vi "PID Intake.vi"(8 "Cluster 3":T2={"Left Encoder"="Talon1", "Right Encoder"="Talon4", "Gyro Refnum"="Gyro", "Device Number"=enum."Dev0", "Right Refnum"="Talon5", "Left Refnum"="Talon2", "Right Intake"="Talon9", "Left Intake"="Talon7"}, 9 "Timeout":i16, 10 "Target Distance":dbl format="%#_13g", 11 "Target Angle":dbl) -> (0 "Cluster 2":T2={"Left Encoder"="Talon1", "Right Encoder"="Talon4", "Gyro Refnum"="Gyro", "Device Number"=enum."Dev0", "Right Refnum"="Talon5", "Left Refnum"="Talon2", "Right Intake"="Talon9", "Left Intake"="Talon7"})   [LabVIEW 2017]
uses:
  <vilib>/Rock Robotics/WPI/ThirdParty/Sensors/navX/_TypeDefs/FRIC_navX_DeviceNumbersTypeDef.ctl
  Public/Documents/Cross The Road Electronics/Phoenix-LabVIEW/Motor Controller/Controls/CTRE_Phoenix_MotorControl_ControlMode.ctl
  <vilib>/Rock Robotics/WPI/ThirdParty/Phoenix-LabVIEW/Motor Controller/Get/CTRE_Phoenix_MotorController_GetQuadratureData.vi
  <vilib>/addons/control/pid/pid.llb/PID (DBL).vi
  <vilib>/addons/control/pid/NI_PID_pid.lvlib
panel:
  out "In Range":dbl
  out "A-Setpoint":dbl
  in  "D - Lower Limit":dbl=-0.7 format="%#_13g"
  in  "D - Upper Limit":dbl=0.7 format="%#_13g"
  in  "A - Lower Limit":dbl=-1.0 format="%#_13g"
  in  "A - Upper Limit":dbl=1.0 format="%#_13g"
  out "D - Low Threshold":dbl
  out "D - High Threshold":dbl
  out "Cluster":cluster{dbl, dbl}
  out "Angle Modifier":dbl format="%.2f"
  out "Distance Modifier":dbl format="%.2f"
  out "Quadrature Position 4":i32
  out "Quadrature Position 1":i32
  out "Elapsed Time":u32
  out "Distance":i32
  out "Angle":dbl
  in  "A-D":dbl=0.001 format="%#_13g"
  in  "A-I":dbl format="%#_13g"
  in  "A-P":dbl=0.075 format="%#_13g"
  out "Right":dbl
  out "Left":dbl
  in  "D-P":dbl=5e-05 format="%#_13g"
  in  "D-I":dbl format="%#_13g"
  in  "D-D":dbl=1e-07 format="%#_13g"
  out "error out":errorcluster
  in  "error in":errorcluster
  # "pos 1-pos8=distance"
  # "Miami Valley\nDistance\n3E-5\n0\n.001\n.7\n-.7\n\nAngle\n.075\n0\n0\n.5\n-.5\n\n25k=20\" 20.25\"\n50k=39.75\"\n100k=78.5\"\n150k=116.5"
  # ".0002"
  # "4"
  # "2.5E-5"
  # "ALPHA encoders\nTalon1\nTalon4\n\nALPHA drive\nTalon2\nTalon5"
  # ".00001"
  # ".0005"
  # "8e-5/0/1e-7"
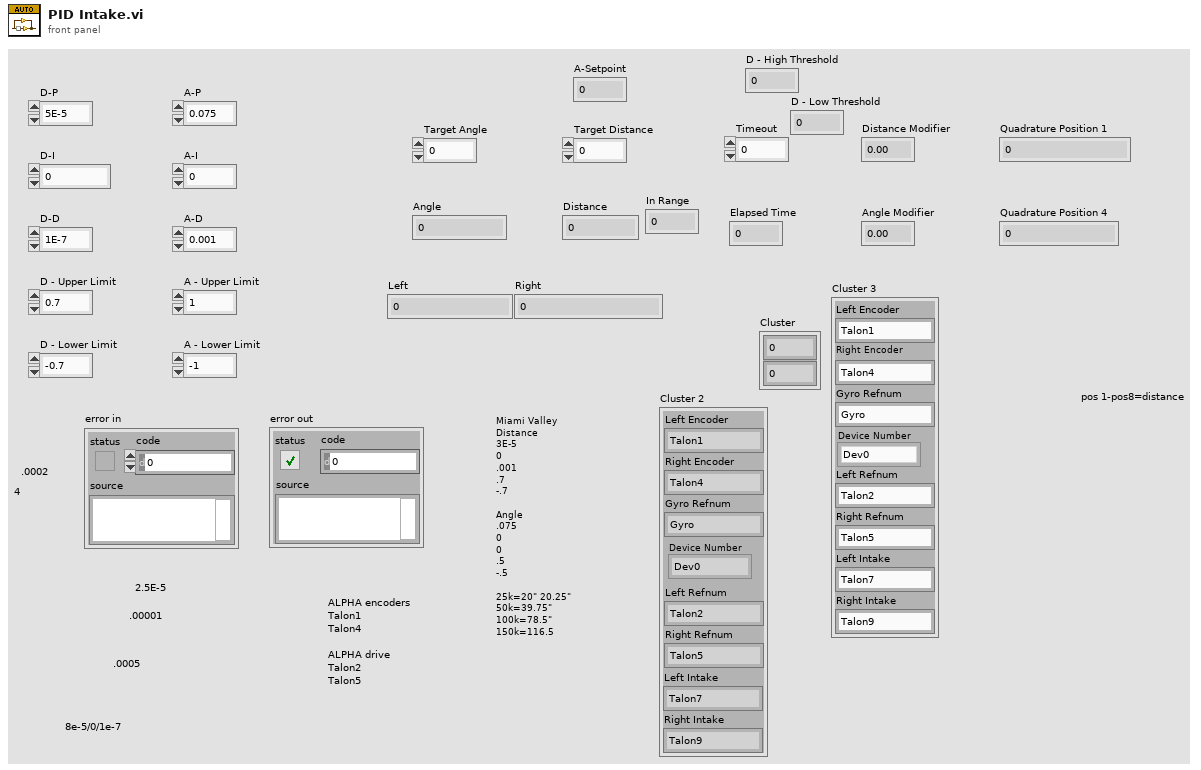
[diagram p1: front panel]
types:
  T1 = typedef "FRIC_navX_DeviceNumbersTypeDef.ctl" = enum16{"Dev0", "Dev1", "Dev2", "Dev3"}
  T2 = cluster{"Left Encoder":string, "Right Encoder":string, "Gyro Refnum":string, "Device Number":T1, "Right Refnum":string, "Left Refnum":string, "Right Intake":string, "Left Intake":string}
  T3 = typedef "CTRE_Phoenix_MotorControl_ControlMode.ctl" = u16
  T4 = typedef "WPI_GyroDevRef.ctl" = cluster{"DevStatus":errorcluster, "Analog Channel":T5, "Gain (VoltsPerDegree/Second)":dbl, "Gyro Type":enum16{"Analog", "XRS450"}, "Handle":i32, "SPI Bus":T6, "Device Found":bool, "Sample Rate":dbl, "Calibrate On Open":bool, "Offset":dbl}
  T5 = typedef "FPGA_AIChannel.ctl" = enum8{"AI 0", "AI 1", "AI 2", "AI 3", "AI MXP 0", "AI MXP 1", "AI MXP 2", "AI MXP 3", "Invalid"}
  T6 = typedef "spi_bus.ctl" = enum16{"SPI On-Board, CS0", "SPI On-Board, CS1", "SPI On-Board, CS2", "SPI On-Board, CS3", "SPI MXP", "Invalid"}
  T7 = typedef "WPI_MotorControlDeviceRef.ctl" = cluster{"DeviceStatus":errorcluster, "Type":T8, "PWM":cluster{"PWM Channel":T9, "DeadBand":T10}, "CAN":cluster{"Device Number":u8, "SetOutput VI Ref":variant, "GetOutput VI Ref":variant, "Enable VI Ref":variant, "Disable VI Ref":variant, "Data":variant}, "Invert":bool, "DIO PWM":cluster{"PWM \"Enable\" Channel":T9, "DIOChannel":T11, "PWM Rate":dbl}}
  T8 = typedef "WPI_MotorControlType.ctl" = enum16{"PWM", "CAN", "DIO PWM"}
  T9 = typedef "FPGA_DIOPWMChannel.ctl" = enum8{"PWM 0", "PWM 1", "PWM 2", "PWM 3", "PWM 4", "PWM 5", "PWM 6", "PWM 7", "PWM 8", "PWM 9", "PWM MXP 0", "PWM MXP 1", "PWM MXP 2", "PWM MXP 3", "PWM MXP 4", "PWM MXP 5", "PWM MXP 6", "PWM MXP 7", "PWM MXP 8", "PWM MXP 9", "Invalid"}
  T10 = typedef "WPI_PWMDeadband.ctl" = cluster{"Name":string, "maxPositivePwm":i32, "minPositivePwm":i32, "centerPwm":i32, "maxNegativePwm":i32, "minNegativePwm":i32, "angularRange":u16}
  T11 = typedef "FPGA_DIOChannel.ctl" = enum8{"DIO 0", "DIO 1", "DIO 2", "DIO 3", "DIO 4", "DIO 5", "DIO 6", "DIO 7", "DIO 8", "DIO 9", "DIO MXP 0", "DIO MXP 1", "DIO MXP 2", "DIO MXP 3", "DIO MXP 4", "DIO MXP 5", "DIO MXP 6", "DIO MXP 7", "DIO MXP 8", "DIO MXP 9", "DIO MXP 10", "DIO MXP 11", "DIO MXP 12", "DIO MXP 13", "DIO MXP 14", "DIO MXP 15", "SPI Port CS1", "SPI Port CS2", "SPI Port CS3", "SPI Port MISO", "SPI Port MOSI", "Invalid"}
  T12 = cluster{"D - Upper Limit":dbl, "D - Lower Limit":dbl}
  T13 = cluster{"A - Upper Limit":dbl, "A - Lower Limit":dbl}
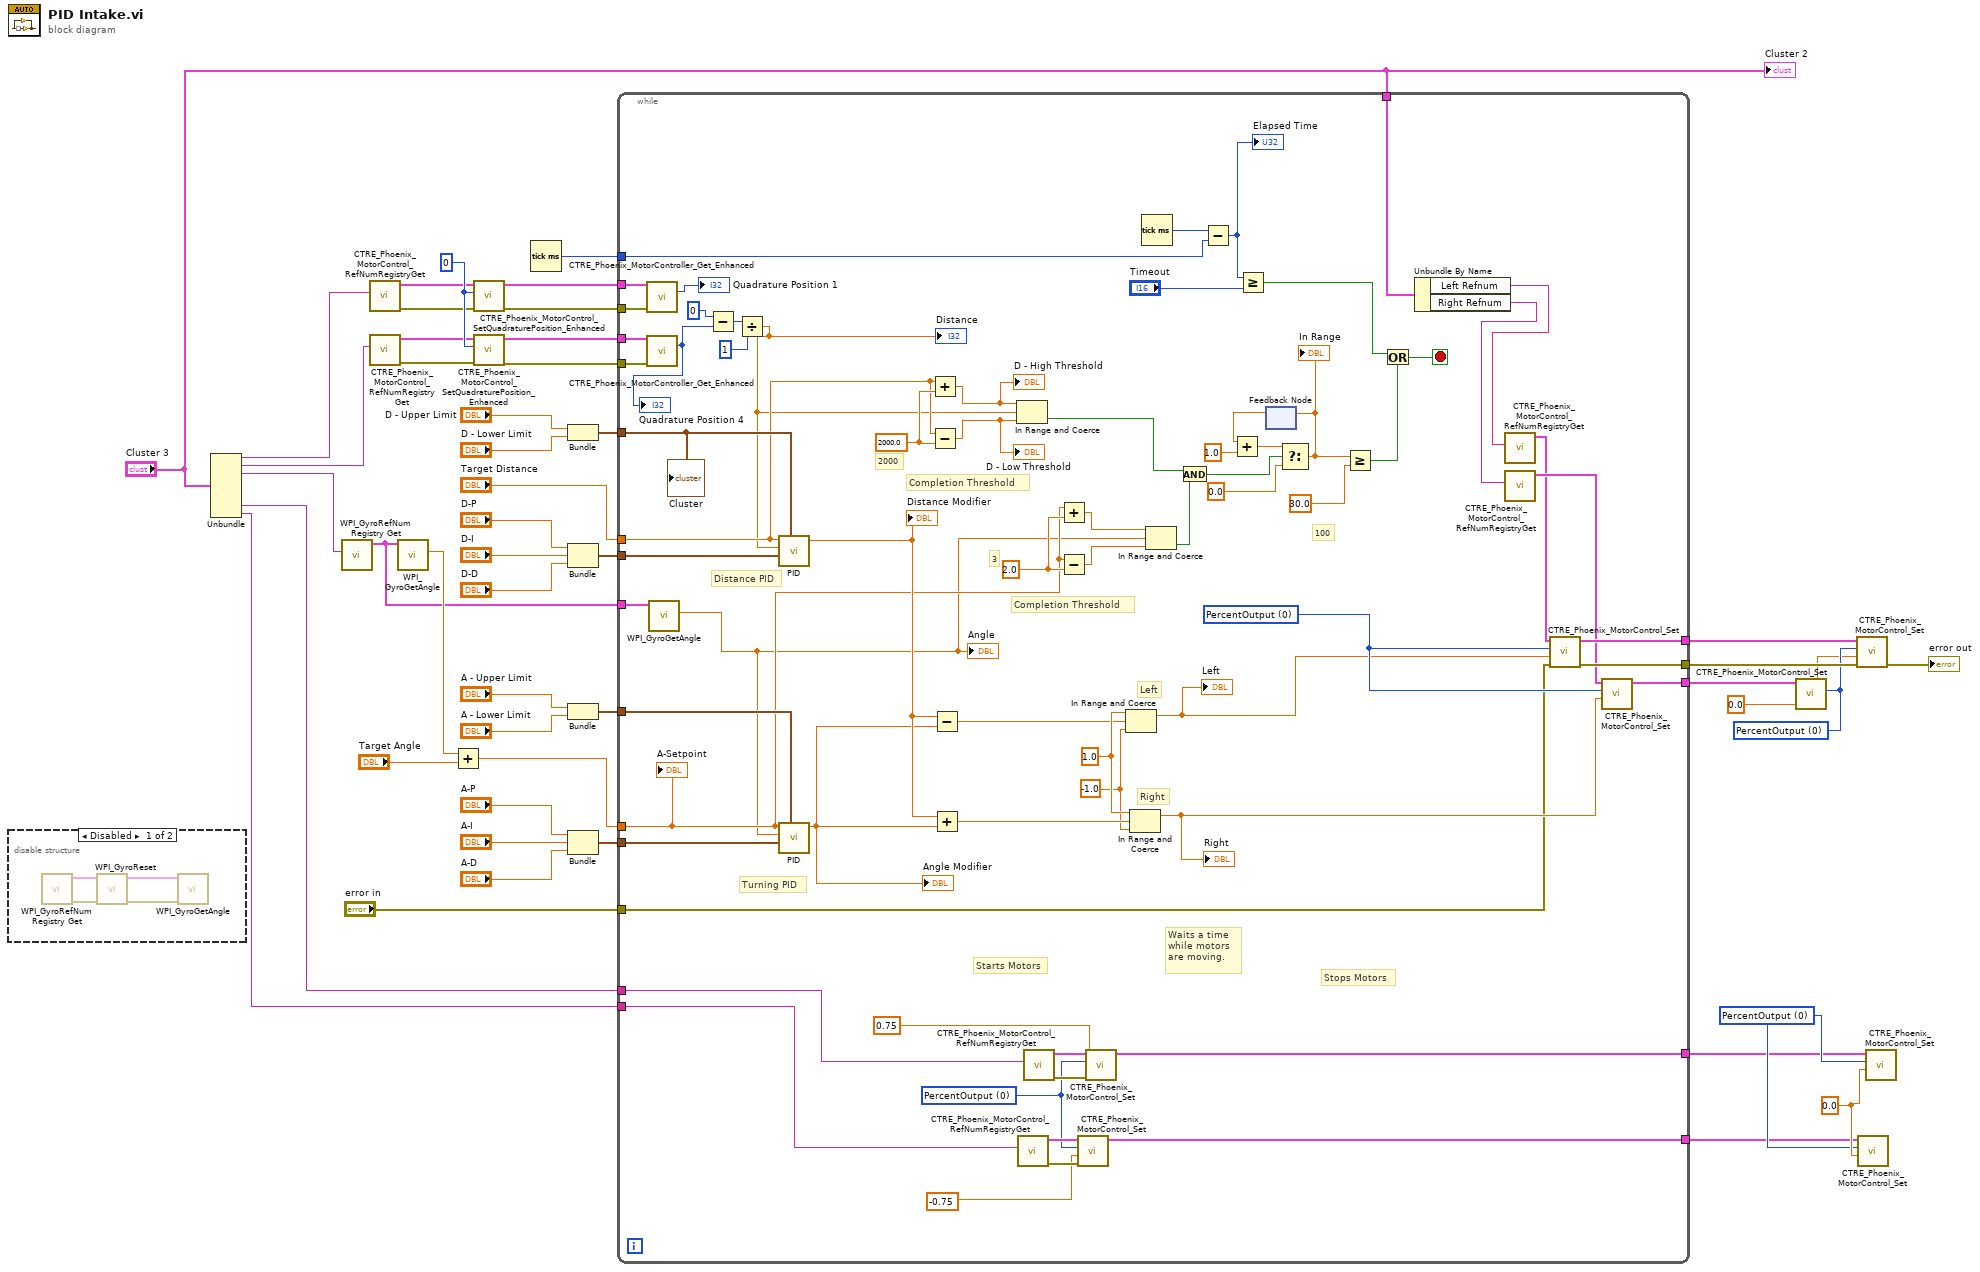
[diagram p0: block diagram]
diagram:
  w4 = 0.0 ("Output")
  w3 = T3 0 items=["PercentOutput"=0, "Position"=1, "Velocity"=2, "Current"=3, "Follower"=5, "MotionProfile"=6, "MotionMagic"=7, "MotionMagicArc"=8, "MotionProfileArc"=10, "Disabled"=15] ("Control Mode")
  w9 = 0.0 ("Output")
  w10 = T3 0 items=["PercentOutput"=0, "Position"=1, "Velocity"=2, "Current"=3, "Follower"=5, "MotionProfile"=6, "MotionMagic"=7, "MotionMagicArc"=8, "MotionProfileArc"=10, "Disabled"=15] ("Control Mode")
  w29 = 0 ("New Position")
  n1 = disable-structure shown="Disabled" {
    frame Disabled {
      n2 = call <vilib>:"WPI_GyroRefNum Registry Get.vi"() -> ("error out"=w49:errorcluster, "GyroDevRef"=w50:T4)  [unwired: 10 in]
      n3 = call <vilib>:"WPI_GyroReset.vi"("error in"=w49, "GyroDevRef"=w50) -> ("error out"=w47:errorcluster, "GyroDevRef"=w48:T4)  [unwired: 8 in]
      n4 = call <vilib>:"WPI_GyroGetAngle.vi"("error in"=w47, "GyroDevRef"=w48) -> ()  [unwired: 5 in, 5 out]
    }
    frame Enabled {
    }
  }
  n5 = Unbundle("Cluster 3") -> ("Left Encoder"=w23:string, "Right Encoder"=w22:string, "Gyro Refnum"=w19:string, "Right Intake"=w6:string, "Left Intake"=w5:string)  [unwired: 3 out]
  n6 = call <vilib>:"WPI_GyroRefNum Registry Get.vi"("refnum name"=w19) -> ("GyroDevRef"=w17:T4)  [unwired: 9 in, 1 out]
  n7 = call "CTRE_Phoenix_MotorControl_RefNumRegistryGet.vi"("refnum name"=w23) -> ("error out"=w25:errorcluster, "PhoenixMotorControlDevRef"=w16:T7)  [unwired: 9 in]
  n8 = call "CTRE_Phoenix_MotorControl_RefNumRegistryGet.vi"("refnum name"=w22) -> ("error out"=w27:errorcluster, "PhoenixMotorControlDevRef"=w15:T7)  [unwired: 9 in]
  n9 = call <vilib>:"WPI_GyroGetAngle.vi"("GyroDevRef"=w17) -> ("Angle"=w18:dbl)  [unwired: 6 in, 4 out]
  n10 = Add(x=w18, y="Target Angle") -> (x+y=w20:dbl)
  n11 = call "CTRE_Phoenix_MotorControl_SetQuadraturePosition_Enhanced.vi"("error in (no error)"=w25, "New Position"=w29, "PhoenixMotorControlDevRef"=w16) -> ("error out"=w26:errorcluster, "PhoenixMotorControlDevRef"=w31:T7)  [unwired: 7 in]
  n12 = call "CTRE_Phoenix_MotorControl_SetQuadraturePosition_Enhanced.vi"("error in (no error)"=w27, "New Position"=w29, "PhoenixMotorControlDevRef"=w15) -> ("error out"=w28:errorcluster, "PhoenixMotorControlDevRef"=w30:T7)  [unwired: 7 in]
  n13 = Tick Count (ms)() -> (millisecond timer value=w24:u32)
  n14 = Bundle("D - Upper Limit"="D - Upper Limit", "D - Lower Limit"="D - Lower Limit") -> (w44:T12)  [unwired: 1 in]
  n15 = Bundle("D-P"="D-P", "D-I"="D-I", "D-D"="D-D") -> (w33:cluster{"D-P":dbl, "D-I":dbl, "D-D":dbl})  [unwired: 1 in]
  n16 = Bundle("A - Upper Limit"="A - Upper Limit", "A - Lower Limit"="A - Lower Limit") -> (w41:T13)  [unwired: 1 in]
  n17 = Bundle("A-P"="A-P", "A-I"="A-I", "A-D"="A-D") -> (w37:cluster{"A-P":dbl, "A-I":dbl, "A-D":dbl})  [unwired: 1 in]
  n18 = while {
    tunnel: w44 -> [w119]
    tunnel: w41 -> [w117]
    tunnel: w37 -> [w113]
    tunnel: w33 -> [w112]
    tunnel: "Target Distance" -> [w100]
    tunnel: w20 -> [w93]
    tunnel: w30 -> [w110]
    tunnel: w31 -> [w109]
    tunnel: w28 -> [w108]
    tunnel: w26 -> [w107]
    tunnel: w24 -> [w104]
    tunnel: w17 -> [w83]
    tunnel: [w78] -> w14
    tunnel: [w77] -> w12
    tunnel: [w76] -> w11
    tunnel: "Cluster 3" -> [w75]
    tunnel: "error in" -> [w66]
    tunnel: w6 -> [w56]
    tunnel: w5 -> [w55]
    tunnel: [w52] -> w2
    tunnel: [w51] -> w1
    stop <- w88 stop-if-true
    w57 = T3 0 items=["PercentOutput"=0, "Position"=1, "Velocity"=2, "Current"=3, "Follower"=5, "MotionProfile"=6, "MotionMagic"=7, "MotionMagicArc"=8, "MotionProfileArc"=10, "Disabled"=15] ("Control Mode")
    w67 = -1.0
    w81 = T3 0 items=["PercentOutput"=0, "Position"=1, "Velocity"=2, "Current"=3, "Follower"=5, "MotionProfile"=6, "MotionMagic"=7, "MotionMagicArc"=8, "MotionProfileArc"=10, "Disabled"=15] ("Control Mode")
    w94 = 2.0
    w111 = 2000.0
    w118 = 1.0
    # "Stops Motors"
    # "Waits a time \nwhile motors \nare moving."
    # "Starts Motors"
    # "100"
    # "3"
    # "2000"
    # "Completion Threshold"
    # "Completion Threshold"
    # "Right"
    # "Left"
    # "Turning PID"
    # "Distance PID"
    n19 = call-poly <vilib>:"CTRE_Phoenix_MotorController_Get_Enhanced.vi"("PhoenixMotorControlDevRef"=w109, "error in"=w107) -> ("Quadrature Position"=→"Quadrature Position 1":i32)  [unwired: 10 in, 3 out]
    n20 = call-poly <vilib>:"CTRE_Phoenix_MotorController_Get_Enhanced.vi"("PhoenixMotorControlDevRef"=w110, "error in"=w108) -> ("Quadrature Position"=w63:i32)  [unwired: 10 in, 3 out]
    "Quadrature Position 4" <- w63
    n21 = call <vilib>:"WPI_GyroGetAngle.vi"("GyroDevRef"=w83) -> ("Angle"=w82:dbl)  [unwired: 6 in, 4 out]
    "Angle" <- w82
    n22 = Subtract(x=0, y=w63) -> (x-y=w85:i32)
    n23 = Divide(x=w85, y=1) -> (x/y=w65:dbl)
    "Distance" <- w65
    n24 = call-poly <vilib>:"PID.vi"("output range"=w119, "PID gains"=w112, "process variable"=w65, "setpoint"=w100) -> ("output"=w116:dbl)  [unwired: 6 in, 1 out]
    "Distance Modifier" <- w116
    n25 = call-poly <vilib>:"PID.vi"("output range"=w117, "PID gains"=w113, "process variable"=w82, "setpoint"=w93) -> ("output"=w87:dbl)  [unwired: 6 in, 1 out]
    "Angle Modifier" <- w87
    n26 = Add(x=w100, y=w111) -> (x+y=w99:dbl)
    "D - High Threshold" <- w99
    n27 = Subtract(x=w100, y=w111) -> (x-y=w98:dbl)
    "D - Low Threshold" <- w98
    n28 = Subtract(x=w116, y=w87) -> (x-y=w114:dbl)
    n29 = Add(x=w116, y=w87) -> (x+y=w115:dbl)
    n30 = In Range and Coerce(upper limit=w99, x=w65, lower limit=w98) -> (In Range?=w97:bool)  [unwired: 1 out]
    n31 = call "CTRE_Phoenix_MotorControl_RefNumRegistryGet.vi"("refnum name"=w55) -> ("error out"=w58:errorcluster, "PhoenixMotorControlDevRef"=w59:T7)  [unwired: 9 in]
    n32 = call "CTRE_Phoenix_MotorControl_RefNumRegistryGet.vi"("refnum name"=w56) -> ("error out"=w61:errorcluster, "PhoenixMotorControlDevRef"=w60:T7)  [unwired: 9 in]
    n33 = Add(x=w93, y=w94) -> (x+y=w95:dbl)
    n34 = Subtract(x=w93, y=w94) -> (x-y=w96:dbl)
    n35 = call <vilib>:"CTRE_Phoenix_MotorControl_Set.vi"("error in (no error)"=w58, "Output"=-0.75, "Control Mode"=w57, "PhoenixMotorControlDevRef"=w59) -> ("PhoenixMotorControlDevRef"=w52:T7)  [unwired: 6 in, 1 out]
    n36 = call <vilib>:"CTRE_Phoenix_MotorControl_Set.vi"("error in (no error)"=w61, "Output"=0.75, "Control Mode"=w57, "PhoenixMotorControlDevRef"=w60) -> ("PhoenixMotorControlDevRef"=w51:T7)  [unwired: 6 in, 1 out]
    n37 = In Range and Coerce(upper limit=w118, x=w114, lower limit=w67) -> (coerced(x)=w80:dbl)  [unwired: 1 out]
    "Left" <- w80
    n38 = In Range and Coerce(upper limit=w118, x=w115, lower limit=w67) -> (coerced(x)=w79:dbl)  [unwired: 1 out]
    "Right" <- w79
    n39 = Tick Count (ms)() -> (millisecond timer value=w106:u32)
    n40 = In Range and Coerce(upper limit=w95, x=w82, lower limit=w96) -> (In Range?=w92:bool)  [unwired: 1 out]
    n41 = And(x=w97, y=w92) -> (x .and. y?=w91:bool)
    n42 = Subtract(x=w106, y=w104) -> (x-y=w105:u32)
    "Elapsed Time" <- w105
    n43 = Greater Or Equal?(x=w105, y="Timeout") -> (x >= y?=w90:bool)
    n44 = feedback #1() -> (w102:dbl)  [unwired: 1 in]
    n45 = Add(x=w102, y=1.0) -> (x+y=w103:dbl)
    n46 = Select(t=w103, s=w91, f=0.0) -> (s? t:f=w101:dbl)
    "In Range" <- w101
    n47 = feedback-in #1(w101) -> ()
    n48 = Greater Or Equal?(x=w101, y=30.0) -> (x >= y?=w89:bool)
    n49 = Or(x=w90, y=w89) -> (x .or. y?=w88:bool)
    n50 = Unbundle By Name(w75) -> ("Left Refnum"=w74:string, "Right Refnum"=w73:string)
    n51 = call "CTRE_Phoenix_MotorControl_RefNumRegistryGet.vi"("refnum name"=w74) -> ("PhoenixMotorControlDevRef"=w71:T7)  [unwired: 9 in, 1 out]
    n52 = call "CTRE_Phoenix_MotorControl_RefNumRegistryGet.vi"("refnum name"=w73) -> ("PhoenixMotorControlDevRef"=w72:T7)  [unwired: 9 in, 1 out]
    n53 = call <vilib>:"CTRE_Phoenix_MotorControl_Set.vi"("error in (no error)"=w66, "Output"=w80, "Control Mode"=w81, "PhoenixMotorControlDevRef"=w71) -> ("error out"=w78:errorcluster, "PhoenixMotorControlDevRef"=w77:T7)  [unwired: 6 in]
    n54 = call <vilib>:"CTRE_Phoenix_MotorControl_Set.vi"("Output"=w79, "Control Mode"=w81, "PhoenixMotorControlDevRef"=w72) -> ("PhoenixMotorControlDevRef"=w76:T7)  [unwired: 7 in, 1 out]
    "Cluster" <- w119
    "A-Setpoint" <- w93
  }
  n55 = call <vilib>:"CTRE_Phoenix_MotorControl_Set.vi"("Output"=w9, "Control Mode"=w10, "PhoenixMotorControlDevRef"=w11) -> ()  [unwired: 7 in, 2 out]
  n56 = call <vilib>:"CTRE_Phoenix_MotorControl_Set.vi"("error in (no error)"=w14, "Output"=w9, "Control Mode"=w10, "PhoenixMotorControlDevRef"=w12) -> ("error out"=→"error out":errorcluster)  [unwired: 6 in, 1 out]
  n57 = call <vilib>:"CTRE_Phoenix_MotorControl_Set.vi"("Output"=w4, "Control Mode"=w3, "PhoenixMotorControlDevRef"=w2) -> ()  [unwired: 7 in, 2 out]
  n58 = call <vilib>:"CTRE_Phoenix_MotorControl_Set.vi"("Output"=w4, "Control Mode"=w3, "PhoenixMotorControlDevRef"=w1) -> ()  [unwired: 7 in, 2 out]
  "Cluster 2" <- "Cluster 3"
